vi "RomiSim_Execute_DiffDrive.vi"(7 "out DiffDriveTrainSim in":T1 {"m_Motor"."Jr_KgM2" format="%13.5p"; "m_Motor"."L_H" format="%13.5p"; "m_Motor"."Kt_NMPerAmp" format="%13.5p"; "m_Motor"."KvINV_RadPerSecPerVolt" format="%13.5p"; "m_Motor"."R_Ohms" format="%13.5p"; "m_Motor"."FreeSpeed_RadPerSec" format="%13.5p"; "m_Motor"."FreeCurrent_Amps" format="%13.5p"; "m_Motor"."StallCurrent_Amps" format="%13.5p"; "m_Motor"."StallTorque_NM" format="%13.5p"; "m_Motor"."nominalVoltage_Volts" format="%13.5p"}, 8 "Actual  Battery Voltage":dbl=12.0, 9 "Nominal Battery Voltage":dbl=12.0, 10 "Right Motor Dmd":dbl, 11 "Left Motor Dmd":dbl) -> (1 "Current Amps":dbl, 2 "Battery Volts":dbl, 3 "out DiffDriveTrainSim out":T1 {"m_Motor"."Jr_KgM2" format="%13.5p"; "m_Motor"."L_H" format="%13.5p"; "m_Motor"."Kt_NMPerAmp" format="%13.5p"; "m_Motor"."KvINV_RadPerSecPerVolt" format="%13.5p"; "m_Motor"."R_Ohms" format="%13.5p"; "m_Motor"."FreeSpeed_RadPerSec" format="%13.5p"; "m_Motor"."FreeCurrent_Amps" format="%13.5p"; "m_Motor"."StallCurrent_Amps" format="%13.5p"; "m_Motor"."StallTorque_NM" format="%13.5p"; "m_Motor"."nominalVoltage_Volts" format="%13.5p"})   [LabVIEW 2019]
uses:
  <vilib>/Rock Robotics/WPI/ThirdParty/JAS_Junk/TrajLib/Trajectory_Library.lvlib
  <vilib>/Analysis/Matrix/Datatypes/RealMatrix.ctl
  <vilib>/Analysis/Matrix/NI_Matrix.lvlib
  <vilib>/Rock Robotics/WPI/ThirdParty/JAS_Junk/TrajLib/TypeDef/LINEAR_SYSTEM.ctl
  <vilib>/Rock Robotics/WPI/ThirdParty/JAS_Junk/TrajLib/TypeDef/DCMOTOR.CTL
  <vilib>/Rock Robotics/WPI/ThirdParty/JAS_Junk/TrajLib/TypeDef/DIFF_DRIVE_TRAIN_SIM.ctl
panel:
  # "<States, 1>"
  # "<Outputs, 1>"
  # "<Inputs, 1>"
  # "<Outputs, 1>"
  # "<States,States>"
  # "<States,Inputs>"
  # "<Outputs,States>"
  # "<Outputs,Inputs>"
  # "<States, 1>"
  # "<Outputs, 1>"
  # "<Inputs, 1>"
  # "<Outputs, 1>"
  # "<States,States>"
  # "<States,Inputs>"
  # "<Outputs,States>"
  # "<Outputs,Inputs>"
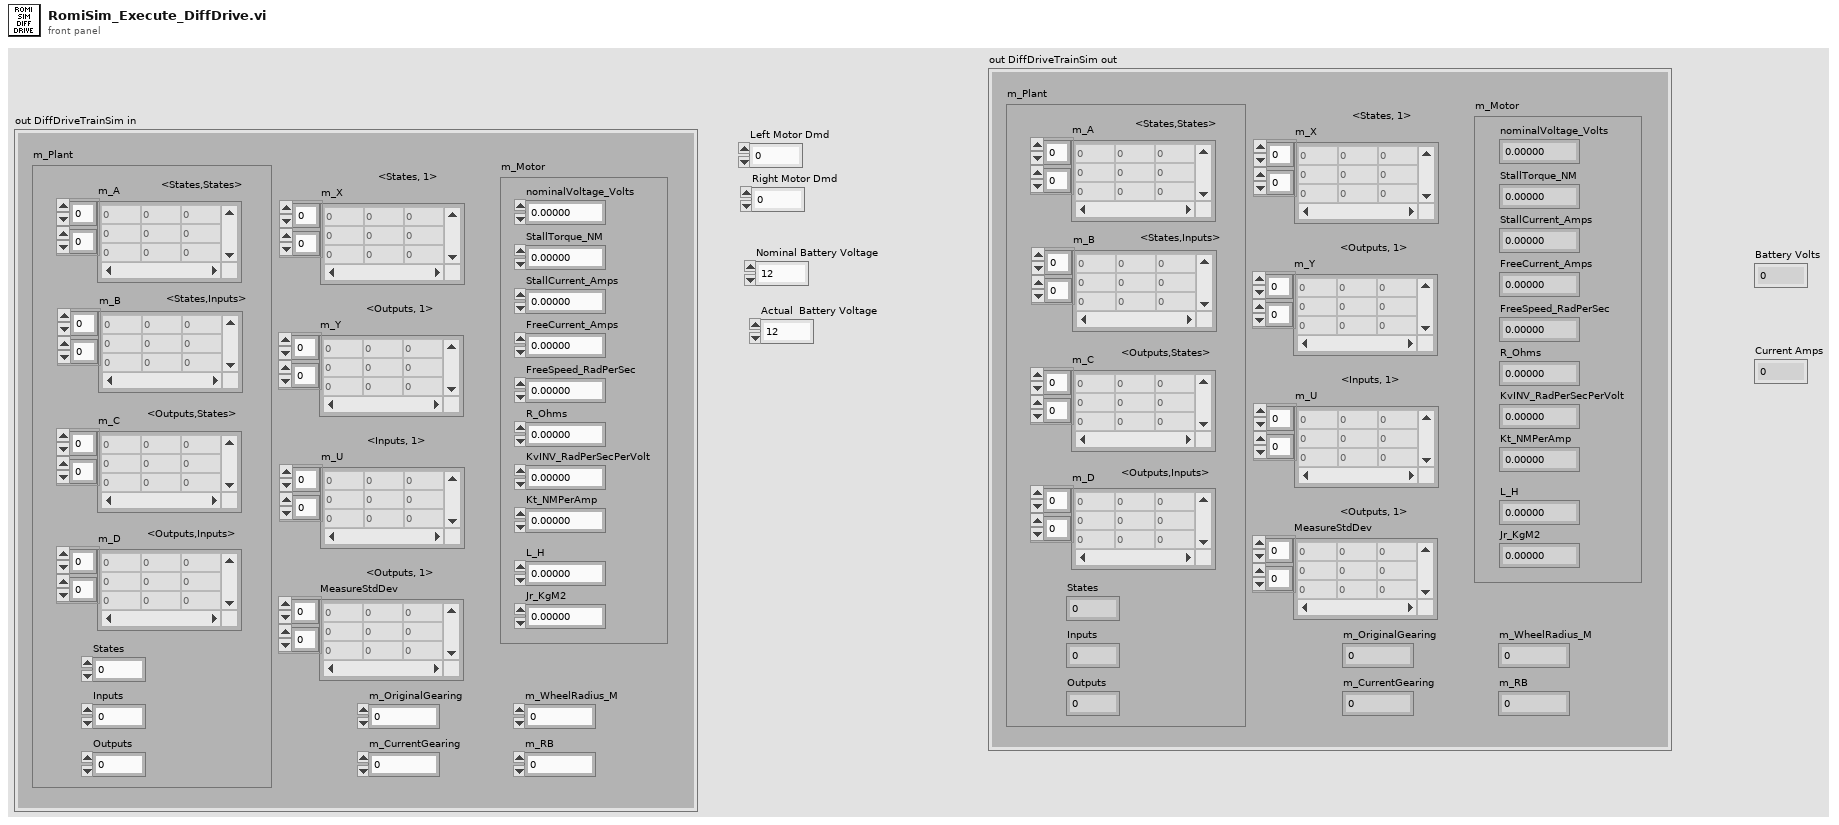
[diagram p1: front panel]
types:
  T1 = typedef "Trajectory_Library.lvlib/DIFF_DRIVE_TRAIN_SIM.ctl" = cluster{"m_Plant":T2, "m_X":T3, "m_Y":T3, "m_U":T3, "MeasureStdDev":T3, "m_Motor":T4, "m_OriginalGearing":dbl, "m_CurrentGearing":dbl, "m_WheelRadius_M":dbl, "m_RB":dbl}
  T2 = typedef "Trajectory_Library.lvlib/LINEAR_SYSTEM.ctl" = cluster{"m_A":T3, "m_B":T3, "m_C":T3, "m_D":T3, "States":i32, "Inputs":i32, "Outputs":i32}
  T3 = typedef "NI_Matrix.lvlib/RealMatrix.ctl" = dbl[][]
  T4 = typedef "Trajectory_Library.lvlib/DCMOTOR.CTL" = cluster{"nominalVoltage_Volts":dbl, "StallTorque_NM":dbl, "StallCurrent_Amps":dbl, "FreeCurrent_Amps":dbl, "FreeSpeed_RadPerSec":dbl, "R_Ohms":dbl, "KvINV_RadPerSecPerVolt":dbl, "Kt_NMPerAmp":dbl, "L_H":dbl, "Jr_KgM2":dbl}
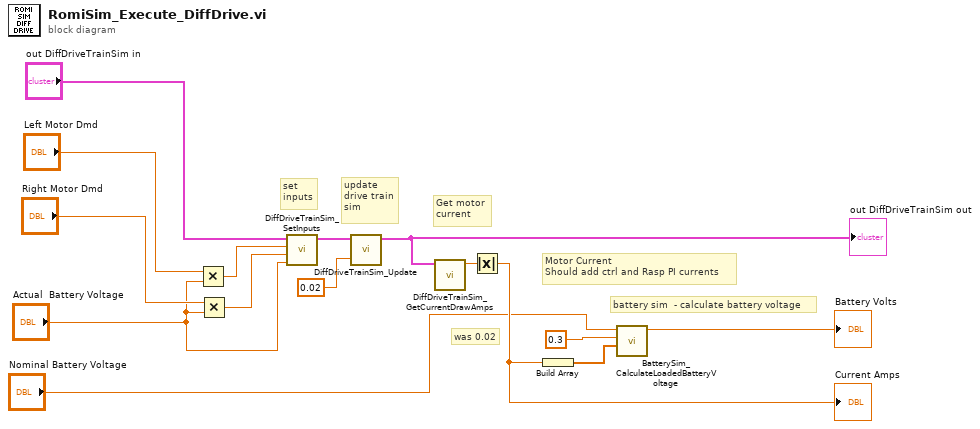
[diagram p0: block diagram]
diagram:
  # "was 0.02"
  # "Get motor\ncurrent"
  # "Motor Current\nShould add ctrl and Rasp PI currents"
  # "update\ndrive train\nsim"
  # "set\ninputs"
  # "battery sim  - calculate battery voltage"
  n1 = Multiply(x="Left Motor Dmd", y="Actual  Battery Voltage") -> (x*y=w12:dbl)
  n2 = Multiply(x="Right Motor Dmd", y="Actual  Battery Voltage") -> (x*y=w13:dbl)
  n3 = call <vilib>:"DiffDriveTrainSim_SetInputs.vi"("BatteryVoltage"="Actual  Battery Voltage", "Right_Volts"=w13, "Left_Volts"=w12, "in DiffDriveTrainSim"="out DiffDriveTrainSim in") -> ("out DiffDriveTrainSim"=w6:T1)  [unwired: 6 in, 1 out]
  n4 = call <vilib>:"DiffDriveTrainSim_Update.vi"("dT_Seconds"=0.02, "in DiffDriveTrainSim"=w6) -> ("out DiffDriveTrainSim"=w3:T1)  [unwired: 8 in, 1 out]
  "out DiffDriveTrainSim out" <- w3
  n5 = call <vilib>:"DiffDriveTrainSim_GetCurrentDrawAmps.vi"("DiffDriveTrainSim"=w3) -> ("TotalCurrent_Amps"=w10:dbl)  [unwired: 10 in]
  n6 = Absolute Value(x=w10) -> (abs(x)=w11:dbl)
  "Current Amps" <- w11
  n7 = Build Array(w11) -> (w9:dbl[])
  n8 = call <vilib>:"BatterySim_CalculateLoadedBatteryVoltage.vi"("Currents"=w9, "Resistance_Ohms"=0.3, "NominalVoltage"="Nominal Battery Voltage") -> ("Voltage"=→"Battery Volts":dbl)  [unwired: 8 in]
